vi "2023 Set Arm Setpoint.vi"(1 "error in (no error)":errorcluster, 2 "armSensorPosition":dbl) -> (0 "error out":errorcluster)   [LabVIEW 2020]
uses:
  2023 Robot Global Data.vi
panel:
  out "armSetpoint":dbl
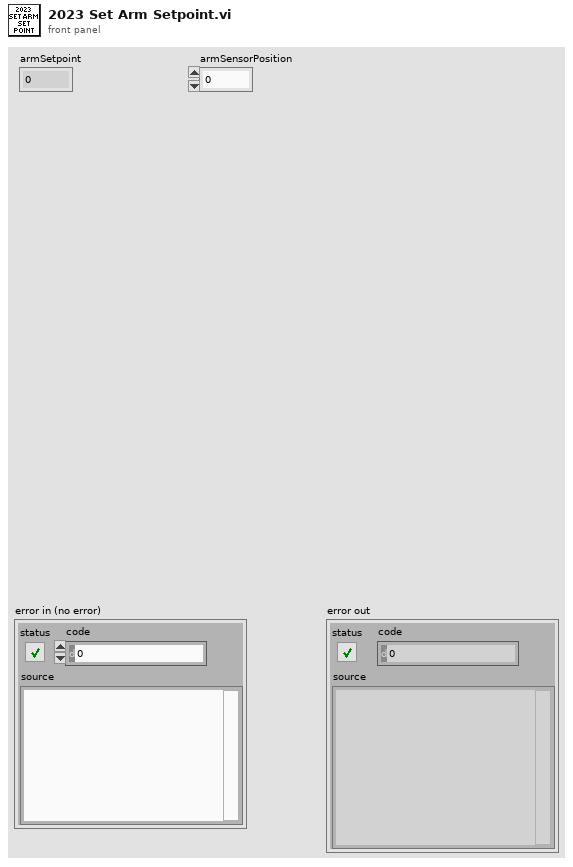
[diagram p1: front panel]
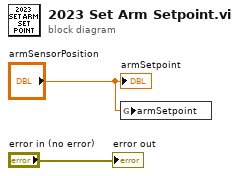
[diagram p0: block diagram]
diagram:
  n1 = global write "2023 Robot Global Data.vi" "armSetpoint"("armSensorPosition") -> ()
  "error out" <- "error in (no error)"
  "armSetpoint" <- "armSensorPosition"
